vi "Experiment.vi"() -> ()   [LabVIEW 2015]
panel:
  out "Array 7":bool[][](array[boolean])
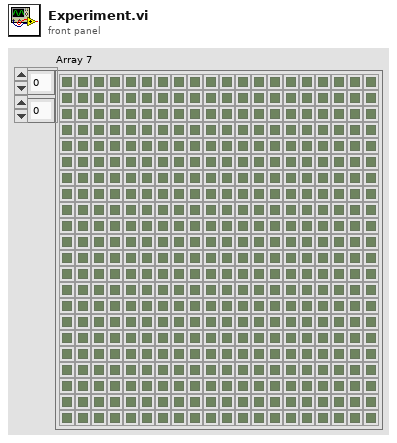
[diagram p1: front panel]
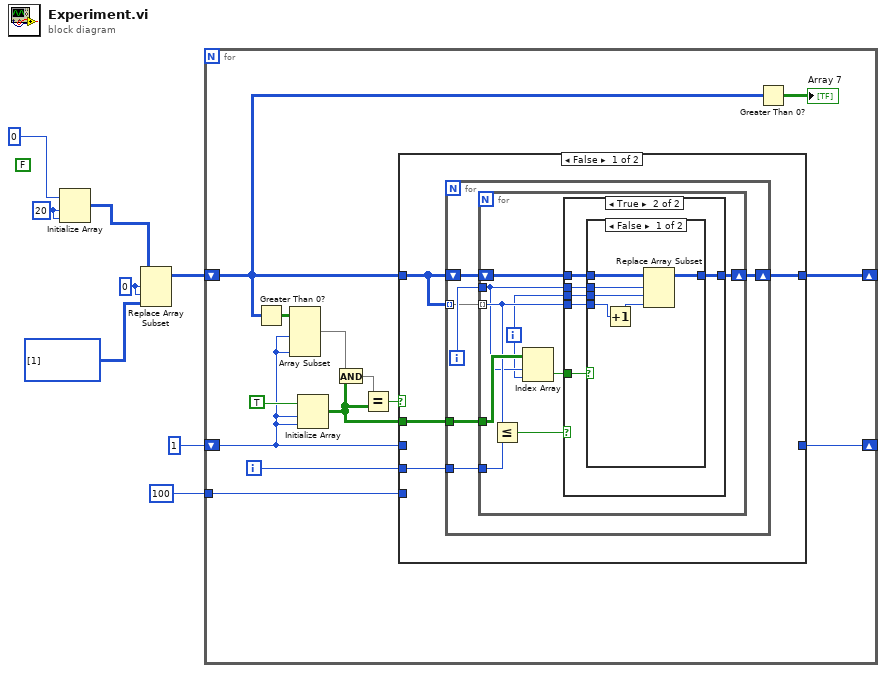
[diagram p0: block diagram]
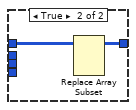
[diagram p3: hidden frame]
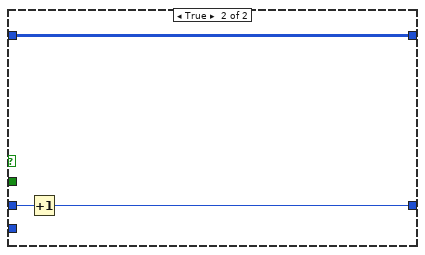
[diagram p4: hidden frame]
diagram:
  w5 = 0 ("index (row)")
  (unwired) FALSE
  w8 = 20 ("dimension size")
  n1 = Initialize Array(0, w8, w8) -> (w7:i32[][])
  n2 = Replace Array Subset(array=w7, new element=i32[][] [[1]] ("initialized array"), index (row)=w5, index (col)=w5) -> (w6:i32[][])
  n3 = for {
    shift-right: [w11] -> _
    shift-left: w6 -> [w10]
    shift-right: [w14] -> _
    shift-left: 1 -> [w15]
    tunnel: 100 -> [w12]
    i -> [w13]
    n4 = Greater Than 0?(x=w10) -> (x > 0?=w19:bool[][])
    n5 = Array Subset(array=w19, length (row)=w15, length (col)=w15) -> (w18:bool[][])  [unwired: 2 in]
    n6 = Initialize Array(TRUE, w15, w15) -> (w9:bool[][])
    n7 = And(x=w18, y=w9) -> (x .and. y?=w17:bool[][])
    n8 = Equal?(x=w17, y=w9) -> (x = y?=w16:bool)
    n9 = case shown="False" w16 {
      tunnel: w15 -> [_ w58]
      tunnel: [_ w57] -> w14
      tunnel: w10 -> [w23 w56]
      tunnel: w13 -> [w24 _]
      tunnel: w12 -> [_ _]
      tunnel: [w22 w56] -> w11
      tunnel: w9 -> [w25 _]
      frame False {
        n10 = for {
          tunnel: w25 -> [w30]
          tunnel: w24 -> [w28]
          shift-right: [w26] -> w22
          shift-left: w23 -> [w31]
          tunnel: w23 -> [w27] mode=indexing
          i -> [w29]
          n11 = for {
            tunnel: w30 -> [w40]
            tunnel: w29 -> [w33]
            tunnel: w28 -> [w39]
            shift-right: [w36] -> w26
            shift-left: w31 -> [w37]
            tunnel: w27 -> [w34] mode=indexing
            i -> [w32]
            n12 = Less Or Equal?(x=w34, y=w39) -> (x <= y?=w38:bool)
            n13 = Index Array(array=w40, index (row)=w33, index (col)=w32) -> (element=w35:bool)
            n14 = case shown="True" w38 {
              tunnel: w37 -> [w41 w47]
              tunnel: [w41 w46] -> w36
              tunnel: w35 -> [_ w45]
              tunnel: w34 -> [_ w44]
              tunnel: w33 -> [_ w43]
              tunnel: w32 -> [_ w42]
              frame False {
              }
              frame True {
                n15 = case shown="False" w45 {
                  tunnel: w47 -> [w53 w55]
                  tunnel: [w52 w54] -> w46
                  tunnel: w44 -> [w49 _]
                  tunnel: w43 -> [w51 _]
                  tunnel: w42 -> [w50 _]
                  frame False {
                    n16 = Increment(x=w49) -> (x+1=w48:i32)
                    n17 = Replace Array Subset(array=w53, new element=w48, index (row)=w51, index (col)=w50) -> (w52:i32[][])
                  }
                  frame True {
                    n18 = Replace Array Subset(array=w55) -> (w54:i32[][])  [unwired: 3 in]
                  }
                }
              }
            }
          }
        }
      }
      frame True {
        n19 = Increment(x=w58) -> (x+1=w57:i32)
      }
    }
    n20 = Greater Than 0?(x=w10) -> (x > 0?=→"Array 7":bool[][])
  }
